vi "Get Module Reconfig Settings.vi"(8 "error in (no error)":errorcluster, 10 "ECAT Mod Reconfig in":T1[](array[typedef]), 11 "RSI Module in":T2 {"Module Config Data"."Config Block Data Refs"."Data Reference" format="%.0x"; "CDOutput Data"."BD Refs"."Data Reference" format="%.0x"; "CDInput Data"."BD Refs"."Data Reference" format="%.0x"; "VS ref" format="%.0x"}) -> (0 "error out":errorcluster, 2 "ECAT Mod Reconfig out":T1[](array[typedef]), 3 "RSI Module out":T2 {"Module Config Data"."Config Block Data Refs"."Data Reference" format="%.0x"; "CDOutput Data"."BD Refs"."Data Reference" format="%.0x"; "CDInput Data"."BD Refs"."Data Reference" format="%.0x"; "VS ref" format="%.0x"})   [LabVIEW 2016, in "Scan Engine Custom Device.lvlib"]
uses:
  Scan Engine Custom Device.lvlib
  Type Defs/RSI Module Data.ctl
  <vilib>/NI Veristand/Custom Device API/Custom Device Item Ref.ctl
  Type Defs/Open Module IOVs.ctl
  Modules.lvlibp/RSI Module/RSI Module.lvclass
  Modules.lvlibp/RSI Module/Module Models.ctl
  Modules.lvlibp/RSI Module/Channel Type.ctl
  Type Defs/Input Data.ctl
  <vilib>/NI Veristand/Custom Device API/Block Data Reference.ctl
  <vilib>/NI Veristand/Custom Device API/Data Reference.ctl
  Type Defs/Output Data.ctl
  Type Defs/Module Config Data.ctl
  Type Defs/Mixed IO.ctl
  Type Defs/ECAT Module Reconfig.ctl
  Type Defs/Data Ref FGV Command.ctl
  <vilib>/NI Veristand/Custom Device API/Custom Device Channel Type.ctl
  <vilib>/NI Veristand/Custom Device API/Data Access Type.ctl
  Modules.lvlibp/RSI Module/Channel GUIDs.vi
  <vilib>/NI Veristand/Custom Device Tools/Custom Device Utility Library/NI VeriStand - Search for Item by GUID.vi
  <vilib>/NI Veristand/Custom Device API/Custom Device API.lvlib
  <vilib>/NI Veristand/Custom Device Tools/Custom Device Utility Library/Custom Device Utility Library.lvlib
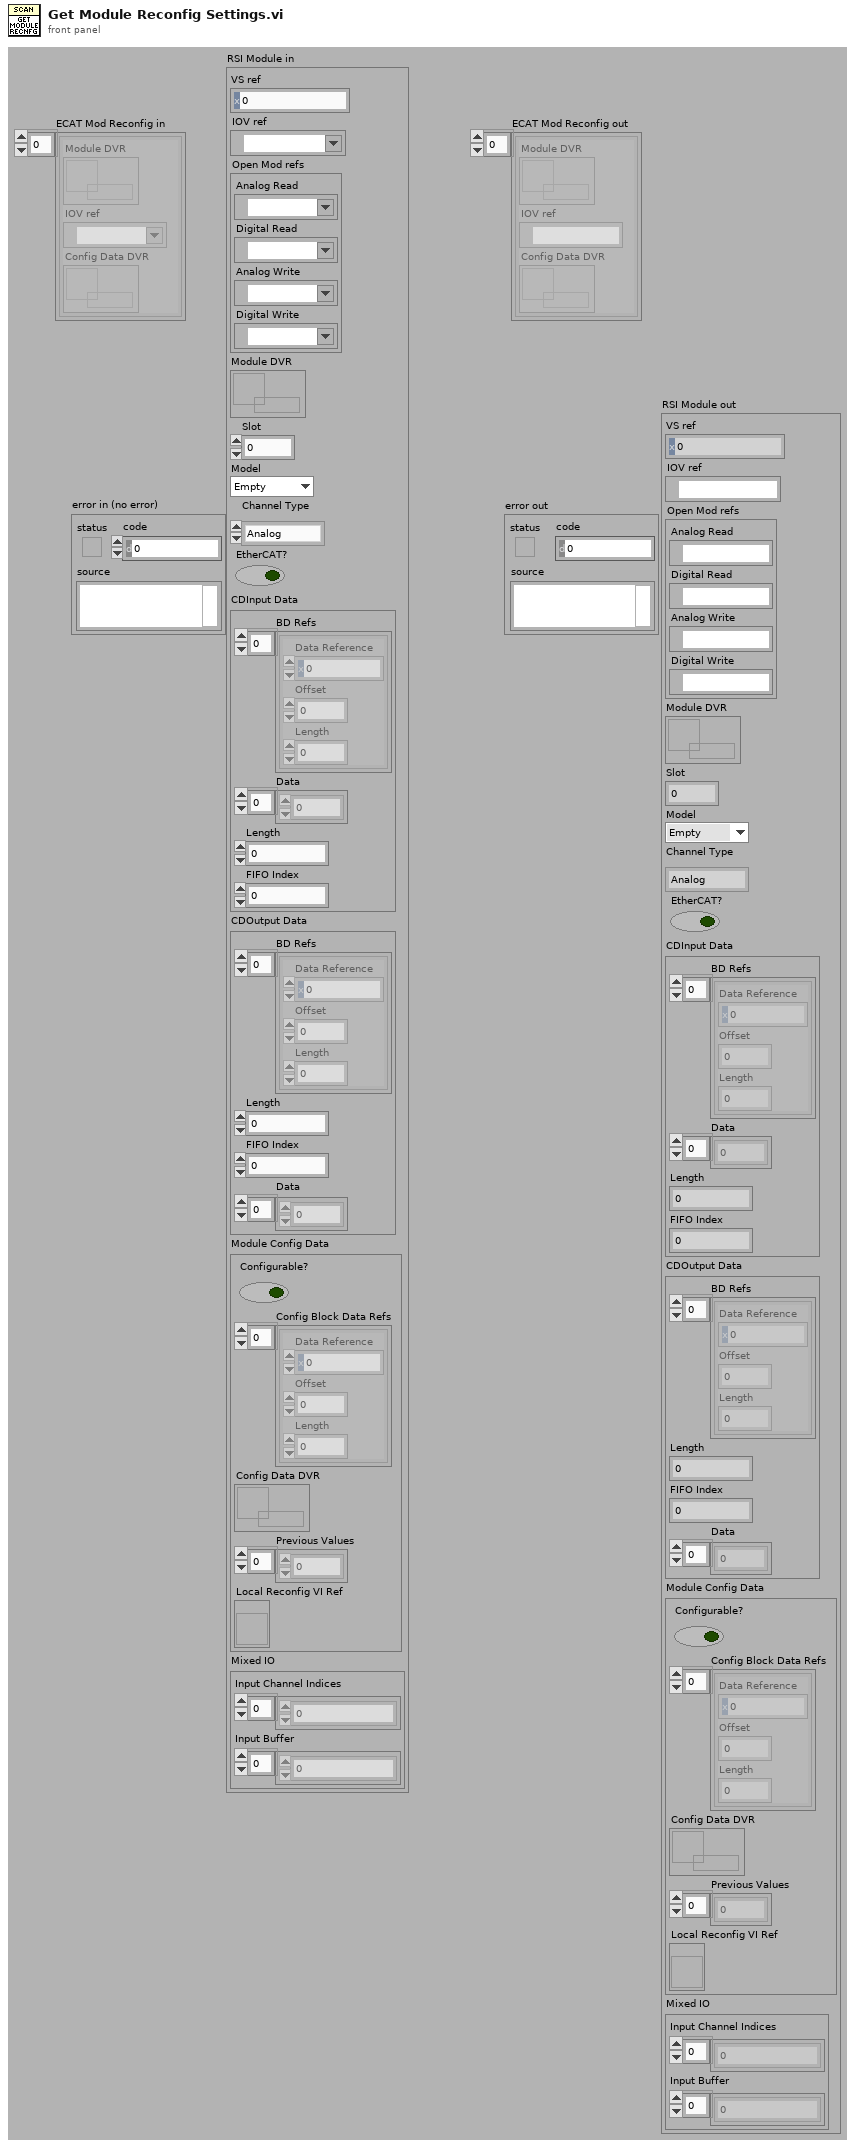
[diagram p1: front panel]
types:
  T1 = typedef "Scan Engine Custom Device.lvlib/ECAT Module Reconfig.ctl" = cluster{"Module DVR":refnum<data-value>, "IOV ref":refnum<k21>, "Config Data DVR":refnum<data-value>}
  T2 = typedef "Scan Engine Custom Device.lvlib/RSI Module Data.ctl" = cluster{"VS ref":T3, "IOV ref":refnum<k21>, "Open Mod refs":T4, "Module DVR":refnum<data-value>, "Slot":u32, "Model":T5, "Channel Type":T6, "EtherCAT?":bool, "CDInput Data":T7, "CDOutput Data":T10, "Module Config Data":T11, "Mixed IO":T12}
  T3 = typedef "Custom Device API.lvlib/Custom Device Item Ref.ctl" = u64
  T4 = typedef "Scan Engine Custom Device.lvlib/Open Module IOVs.ctl" = cluster{"Analog Read":refnum<k21>, "Digital Read":refnum<k21>, "Analog Write":refnum<k21>, "Digital Write":refnum<k21>}
  T5 = typedef "Modules.lvlibp/RSI Module.lvclass/Module Models.ctl" = enum16{"Empty", "NI 9201", "NI 9203", "NI 9205", "NI 9206", "NI 9207", "NI 9208", "NI 9211", "NI 9212", "NI 9213", "NI 9214", "NI 9215", "NI 9217", "NI 9219", "NI 9220", "NI 9221", "NI 9222", "NI 9223", "NI 9225", "NI 9227", "NI 9229", "NI 9233", "NI 9234", "NI 9235", "NI 9236", "NI 9237", "NI 9239", "NI 9242", "NI 9244", "NI 9263", "NI 9264", "NI 9265", "NI 9269", "NI 9375", "NI 9401", "NI 9402", "NI 9403", "NI 9411", "NI 9421", "NI 9422", "NI 9423", "NI 9425", "NI 9426", "NI 9435", "NI 9437", "NI 9472", "NI 9474", "NI 9475", "NI 9476", "NI 9477", "NI 9478", "NI 9481", "NI 9482", "NI 9485"}
  T6 = typedef "Modules.lvlibp/RSI Module.lvclass/Channel Type.ctl" = enum16{"Analog", "Digital"}
  T7 = typedef "Scan Engine Custom Device.lvlib/Input Data.ctl" = cluster{"BD Refs":T8[], "Data":dbl[], "Length":i32, "FIFO Index":i32}
  T8 = typedef "Custom Device API.lvlib/Block Data Reference.ctl" = cluster{"Data Reference":T9, "Offset":u64, "Length":u64}
  T9 = typedef "Custom Device API.lvlib/Data Reference.ctl" = i32
  T10 = typedef "Scan Engine Custom Device.lvlib/Output Data.ctl" = cluster{"BD Refs":T8[], "Length":i32, "FIFO Index":i32, "Data":dbl[]}
  T11 = typedef "Scan Engine Custom Device.lvlib/Module Config Data.ctl" = cluster{"Configurable?":bool, "Config Block Data Refs":T8[], "Config Data DVR":refnum<data-value>, "Previous Values":dbl[], "Local Reconfig VI Ref":refnum<vi>}
  T12 = typedef "Scan Engine Custom Device.lvlib/Mixed IO.ctl" = cluster{"Input Channel Indices":i32[], "Input Buffer":dbl[]}
  T13 = typedef "Custom Device API.lvlib/Data Access Type.ctl" = enum16{"Read", "Write"}
  T14 = typedef "Custom Device API.lvlib/Custom Device Channel Type.ctl" = enum16{"Input", "Output"}
  T15 = typedef "Scan Engine Custom Device.lvlib/Data Ref FGV Command.ctl" = enum16{"Intialize", "Get", "Update"}
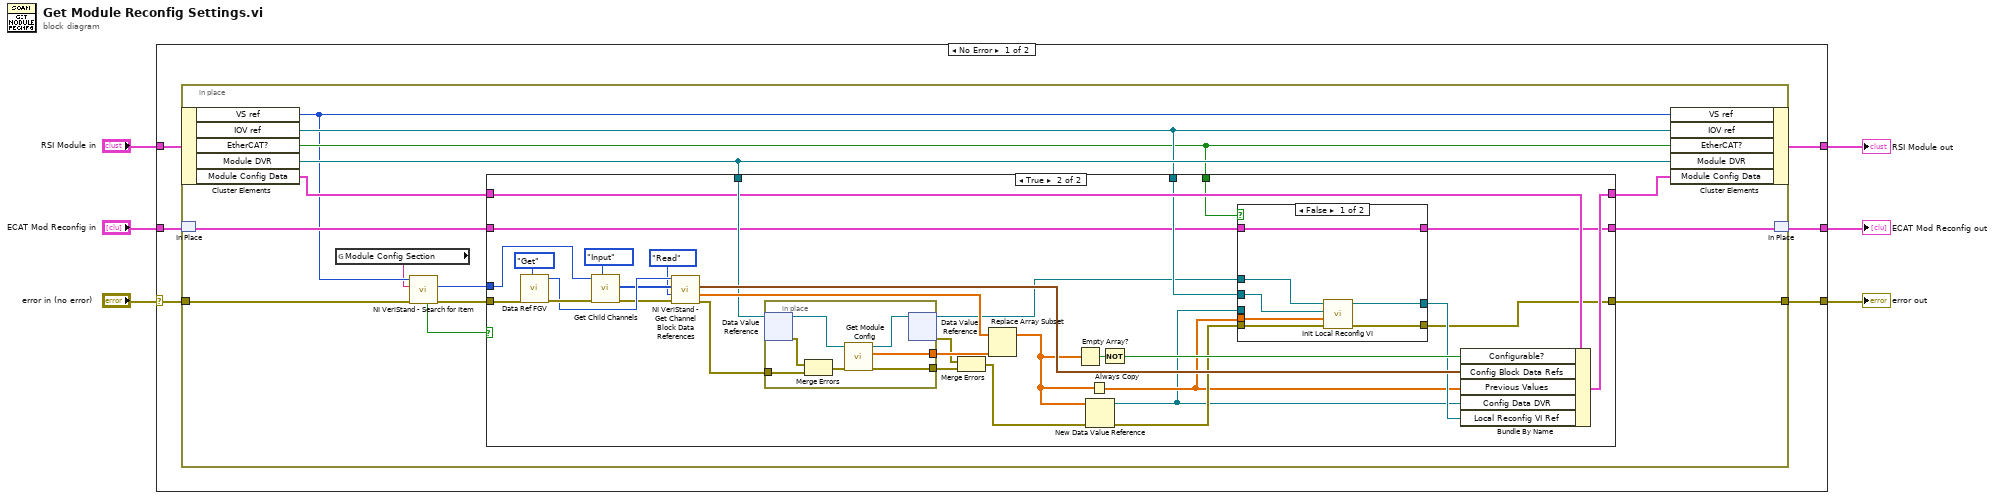
[diagram p0: block diagram]
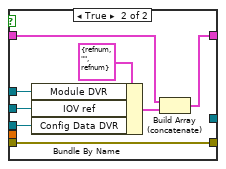
[diagram p3: hidden frame]
diagram:
  n1 = case shown="No Error" "error in (no error)" {
    selector: "error in (no error)" -> [w11 w86]
    tunnel: [w12 w86] -> w5
    tunnel: "RSI Module in" -> [w10 w85]
    tunnel: [w9 w85] -> w3
    tunnel: "ECAT Mod Reconfig in" -> [w8 w84]
    tunnel: [w7 w84] -> w1
    frame No Error {
      n2 = in-place {
        in-place-border: [w26] -> w12
        in-place-border: w11 -> [w18]
        n3 = in-place-cluster #1(w10) -> ("VS ref"=w17:T3, "IOV ref"=w22:refnum<k21>, "EtherCAT?"=w21:bool, "Module DVR"=w24:refnum<data-value>, "Module Config Data"=w23:T11)
        n4 = in-place-match #2(w8) -> (w20:T1[])
        n5 = global read "Channel GUIDs.vi" "Module Config Section"() -> (w16:string)
        n6 = call-poly <vilib>:"NI VeriStand - Search for Item.vi"("error in"=w18, "Item GUID"=w16, "Section Ref in"=w17) -> ("error out"=w14:errorcluster, "Item Ref"=w15:T3, "Found"=w13:bool)  [unwired: 5 in, 1 out]
        n7 = case shown="True" w13 {
          tunnel: [w29 w35] -> w26
          tunnel: [w28 w53] -> w25
          tunnel: w14 -> [w29 w52]
          tunnel: w15 -> [_ w49]
          tunnel: w24 -> [_ w44]
          tunnel: w23 -> [w28 w40]
          tunnel: w22 -> [_ w36]
          tunnel: w21 -> [_ w33]
          tunnel: w20 -> [w27 w31]
          tunnel: [w27 w30] -> w19
          frame False {
          }
          frame True {
            n8 = call "Data Ref FGV.vi"("Command"=Data_Ref_FGV_Command."Get", "error in (no error)"=w52) -> ("error out"=w60:errorcluster, "Device Ref out"=w58:T3)  [unwired: 6 in, 2 out]
            n9 = call "Get Child Channels.vi"("Channel Type"=Custom_Device_Channel_Type."Input", "error in"=w60, "Section Ref in"=w49) -> ("error out"=w56:errorcluster, "Channel Refs"=w57:T3[])  [unwired: 5 in, 2 out]
            n10 = call <vilib>:"NI VeriStand - Get Channel Block Data References.vi"("error in (no error)"=w56, "Access"=Data_Access_Type."Read", "Channel Refs"=w57, "Device Ref in"=w58) -> ("error out"=w47:errorcluster, "Values Array"=w46:dbl[], "Block Data Refs"=w54:T8[])  [unwired: 4 in, 1 out]
            n11 = in-place {
              in-place-border: [w83] -> w48
              in-place-border: w47 -> [w80]
              in-place-border: [w82] -> w43
              n12 = in-place-dvr #3(w44) -> (w78:refnum<class "RSI Module.lvclass">, w81:errorcluster)
              n13 = Merge Errors(w81, w80) -> (w79:errorcluster)
              n14 = call-dynamic "Get Module Config.vi"("error in (no error)"=w79, "RSI Module in"=w78) -> ("error out"=w82:errorcluster, "Config Channels"=w83:dbl[], "RSI Module out"=w77:refnum<class "RSI Module.lvclass">)  [unwired: 7 in]
              n15 = in-place-dvr #3(w77) -> (w34:refnum<data-value>, w42:errorcluster)
            }
            n16 = Merge Errors(w42, w43) -> (w41:errorcluster)
            n17 = Replace Array Subset(array=w46, new element=w48) -> (w45:dbl[])  [unwired: 1 in]
            n18 = Empty Array?(array=w45) -> (empty?=w51:bool)
            n19 = Always Copy(1:w45) -> (0:w37:dbl[])
            n20 = New Data Value Reference(data value=w45, error in=w41) -> (data value reference=w32:refnum<data-value>, error out=w38:errorcluster)
            n21 = Not(x=w51) -> (.not. x?=w50:bool)
            n22 = case shown="False" w33 {
              tunnel: [w68 _] -> w39
              tunnel: w38 -> [w67 w76]
              tunnel: w37 -> [w66 _]
              tunnel: w36 -> [w65 w73]
              tunnel: [w64 w76] -> w35
              tunnel: w34 -> [w63 w74]
              tunnel: w32 -> [_ w72]
              tunnel: w31 -> [w62 w70]
              tunnel: [w62 w71] -> w30
              frame False {
                n23 = call "Init Local Reconfig VI.vi"("error in (no error)"=w67, "Config Channels"=w66, "IOV ref"=w65, "Module DVR"=w63) -> ("error out"=w64:errorcluster, "Local Reconfig VI Ref"=w68:refnum<vi>)  [unwired: 6 in]
              }
              frame True {
                n24 = Bundle By Name(cluster=T1 {"Module DVR"=refnum, "IOV ref"="", "Config Data DVR"=refnum} ("ECAT Module Reconfig"), "Module DVR"=w74, "IOV ref"=w73, "Config Data DVR"=w72) -> (w69:T1)
                n25 = Build Array (concatenate)(w70, w69) -> (w71:T1[])
              }
            }
            n26 = Bundle By Name(cluster=w40, "Configurable?"=w50, "Config Block Data Refs"=w54, "Previous Values"=w37, "Config Data DVR"=w32, "Local Reconfig VI Ref"=w39) -> (w53:T11)
          }
        }
        n27 = in-place-cluster #1("VS ref"=w17, "IOV ref"=w22, "EtherCAT?"=w21, "Module DVR"=w24, "Module Config Data"=w25) -> (w9:T2)
        n28 = in-place-match #2(w19) -> (w7:T1[])
      }
    }
    frame Error {
    }
  }
  "error out" <- w5
  "RSI Module out" <- w3
  "ECAT Mod Reconfig out" <- w1
